vi "Convert Error Code.vi"(9 "Error String":string) -> (1 "VISA Error Code":i32 format="%x")   [LabVIEW 2020, in "Olympus IX BX Series.lvlib"]
doc: "This VI convert Olympus error codes to VISA error codes."
uses:
  Olympus IX BX Series.lvlib
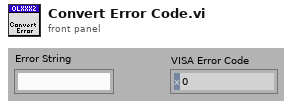
[diagram p1: front panel]
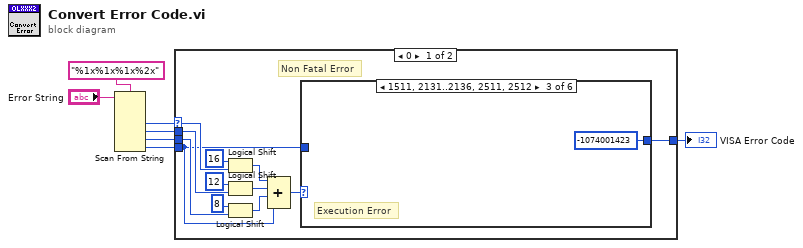
[diagram p0: block diagram]
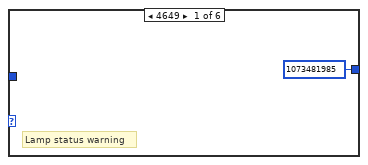
[diagram p2: hidden frame]
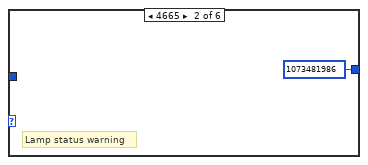
[diagram p3: hidden frame]
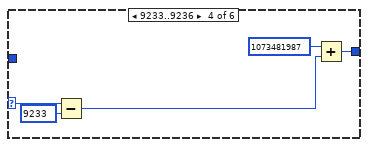
[diagram p4: hidden frame]
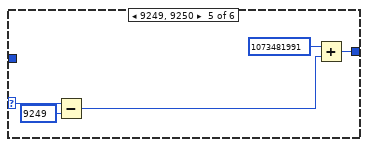
[diagram p5: hidden frame]
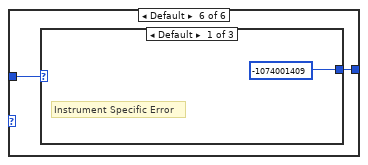
[diagram p6: hidden frame]
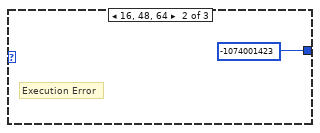
[diagram p7: hidden frame]
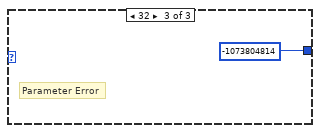
[diagram p8: hidden frame]
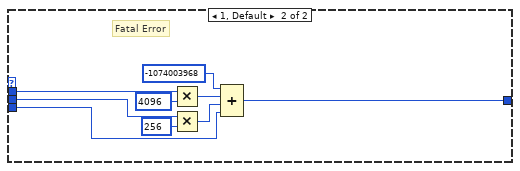
[diagram p9: hidden frame]
diagram:
  n1 = Scan From String(format string="%1x%1x%1x%2x", input string="Error String") -> (output 1=w5:u32, output 2=w4:u32, output 3=w3:u32, output 4=w2:u32)  [unwired: 6 in, 3 out]
  n2 = case shown="0" w5 {
    selector: w5 -> [w17 _]
    tunnel: w4 -> [w16 w45]
    tunnel: w3 -> [w15 w44]
    tunnel: w2 -> [w9 w39]
    tunnel: [w19 w38] -> w1
    frame 0 {
      # "Non Fatal Error"
      n3 = Logical Shift(y=16, x=w17) -> (x << y=w12:u32)
      n4 = Logical Shift(y=12, x=w16) -> (x << y=w11:u32)
      n5 = Logical Shift(y=8, x=w15) -> (x << y=w10:u32)
      n6 = Compound Arithmetic op=ADD(w12, w11, w10, w9) -> (w8:u32)
      n7 = case shown="1511, 2131..2136, 2511, 2512" w8 {
        selector: w8 -> [_ _ _ w27 w32 _]
        tunnel: [1073481985 1073481986 -1074001423 w25 w30 w34] -> w19
        tunnel: w9 -> [_ _ _ _ _ w33]
        frame 4649 {
          # "Lamp status warning"
        }
        frame 4665 {
          # "Lamp status warning"
        }
        frame 5393, 8497..8502, 9489, 9490 {
          # "Execution Error"
        }
        frame 9233..9236 {
          n8 = Subtract(x=w27, y=9233) -> (x-y=w23:u32)
          n9 = Add(x=1073481987, y=w23) -> (x+y=w25:u32)
        }
        frame 9249, 9250 {
          n10 = Subtract(x=w32, y=9249) -> (x-y=w28:u32)
          n11 = Add(x=1073481991, y=w28) -> (x+y=w30:u32)
        }
        frame Default {
          n12 = case shown="Default" w33 {
            tunnel: [-1074001409 -1074001423 -1073804814] -> w34
            frame Default {
              # "Instrument Specific Error"
            }
            frame 16, 48, 64 {
              # "Execution Error"
            }
            frame 32 {
              # "Parameter Error"
            }
          }
        }
      }
    }
    frame 1, Default {
      # "Fatal Error"
      n13 = Multiply(x=w45, y=4096) -> (x*y=w41:u32)
      n14 = Multiply(x=w44, y=256) -> (x*y=w40:u32)
      n15 = Compound Arithmetic op=ADD(-1074003968, w41, w40, w39) -> (w38:u32)
    }
  }
  "VISA Error Code" <- w1
